vi "Shutdown Init.vi"(8 "error in":errorcluster, 11 "SCADA in":refnum<class "EMS.lvclass">) -> (0 "error out":errorcluster, 3 "SCADA out":refnum<class "EMS.lvclass">)   [LabVIEW 2018, in "EMS Core.lvlib" / "EMS.lvclass"]
uses:
  EMS.lvclass
  C:/Program Files (x86)/National Instruments/LabVIEW 2018/vi.lib/ActorFramework/Actor/Actor.lvclass
  Controls/Microgrid State.ctl
  <vilib>/ActorFramework/Time-Delayed Send Message/Time-Delay Override Options.ctl
  EMS.lvclass/EMS.ctl
  <vilib>/ActorFramework/Actor/Actor.lvclass/Actor.ctl
  <vilib>/ActorFramework/Message Enqueuer/Message Enqueuer.lvclass/Message Enqueuer.ctl
  EMS Messages/Return Microgrid State Msg/Return Microgrid State Msg.lvclass/Return Microgrid State Msg.ctl
  <vilib>/ActorFramework/Message Enqueuer/Enqueue.vi
  <vilib>/ActorFramework/Stop Msg/Stop Msg.lvclass
  C:/Program Files (x86)/National Instruments/LabVIEW 2018/vi.lib/ActorFramework/Message/Message.lvclass
  EMS Messages/Return Microgrid State Msg/Return Microgrid State Msg.lvclass
  <vilib>/ActorFramework/Message Priority Queue/Priority Enqueue.vi
  <vilib>/ActorFramework/Actor/Actor.lvclass
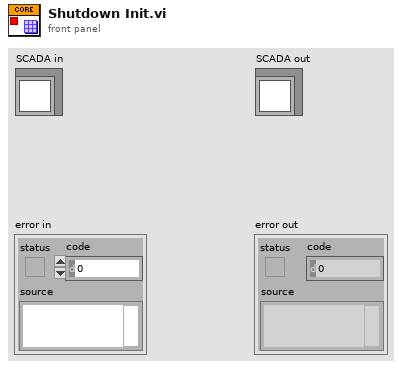
[diagram p1: front panel]
types:
  T1 = typedef "Time-Delay Override Options.ctl" = enum16{"Send next copy now", "Skip next scheduled copy", "Send next copy now and stop all further copies", "Stop all further copies"}
  T2 = typedef "EMS Core.lvlib/EMS.lvclass/Microgrid State.ctl" = enum16{"Discovery", "Commissioning", "Activation", "Blackstart", "OnGrid", "OffGrid", "Island", "Resynchronization", "Manual", "Shutdown", "Stop"}
  T3 = typedef "EMS Core.lvlib/EMS.lvclass/IED Enqueuers.ctl" = cluster{"PV":refnum<class "Message Enqueuer.lvclass">, "IED":refnum<class "Message Enqueuer.lvclass">, "DER":refnum<class "Message Enqueuer.lvclass">, "Relay":refnum<class "Message Enqueuer.lvclass">, "PCC":refnum<class "Message Enqueuer.lvclass">, "ES":refnum<class "Message Enqueuer.lvclass">, "SmartRelay":refnum<class "Message Enqueuer.lvclass">, "ForecastData":refnum<class "Message Enqueuer.lvclass">, "PriceData":refnum<class "Message Enqueuer.lvclass">, "Load":refnum<class "Message Enqueuer.lvclass">, "HVAC":refnum<class "Message Enqueuer.lvclass">, "Meter":refnum<class "Message Enqueuer.lvclass">, "Generator":refnum<class "Message Enqueuer.lvclass">}
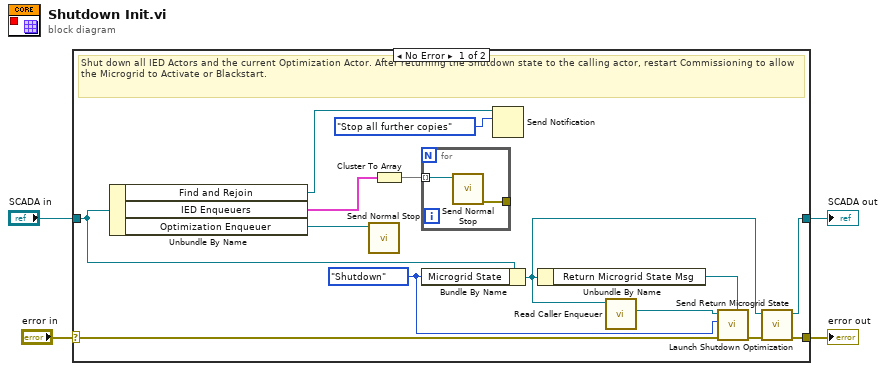
[diagram p0: block diagram]
diagram:
  n1 = case shown="No Error" "error in" {
    selector: "error in" -> [w11 w22]
    tunnel: [w7 w22] -> w3
    tunnel: [w9 w21] -> w1
    tunnel: "SCADA in" -> [w13 w21]
    frame No Error {
      w16 = Microgrid_State."Shutdown" ("Microgrid State")
      # "Shut down all IED Actors and the current Optimization Actor. After returning the Shutdown state to the calling actor, restart Commissioning to allow the Microgrid to Activate or Blackstart."
      n2 = Unbundle By Name(w13) -> ("Find and Rejoin"=w6:refnum<notifier>, "IED Enqueuers"=w15:T3, "Optimization Enqueuer"=w12:refnum<class "Message Enqueuer.lvclass">)
      n3 = call <vilib>:"Send Normal Stop.vi"("Message Enqueuer"=w12) -> ()  [unwired: 10 in, 1 out]
      n4 = Cluster To Array(cluster=w15) -> (array=w14:refnum<class "Message Enqueuer.lvclass">[])
      n5 = for {
        tunnel: w14 -> [w20] mode=indexing
        tunnel: [w19] -> _
        n6 = call <vilib>:"Send Normal Stop.vi"("Message Enqueuer"=w20) -> ("error out"=w19:errorcluster)  [unwired: 10 in]
      }
      n7 = Bundle By Name(cluster=w13, "Microgrid State"=w16) -> (w10:refnum<class "EMS.lvclass">)
      n8 = Send Notification(notification=Time-Delay_Override_Options."Stop all further copies", notifier=w6) -> ()  [unwired: 1 in, 2 out]
      n9 = Unbundle By Name(w10) -> ("Return Microgrid State Msg"=w17:refnum<class "Return Microgrid State Msg.lvclass">)
      n10 = call <vilib>:"Read Caller Enqueuer.vi"("Actor"=w10) -> ("Caller Enqueuer"=w18:refnum<class "Message Enqueuer.lvclass">)  [unwired: 10 in]
      n11 = call "Send Return Microgrid State.vi"("Message Type"=w17, "error in (no error)"=w11, "Microgrid State"=w16, "Message Enqueuer"=w18) -> ("error out"=w8:errorcluster)  [unwired: 6 in, 1 out]
      n12 = call "Launch Shutdown Optimization.vi"("error in"=w8, "SCADA in"=w10) -> ("error out"=w7:errorcluster, "SCADA out"=w9:refnum<class "EMS.lvclass">)  [unwired: 8 in]
    }
    frame Error {
    }
  }
  "error out" <- w3
  "SCADA out" <- w1
